vi "Set BufferLastReadsDBL.vi"(10 "BufferLastReadsDBL.lvclass":refnum<class "BufferLastReadsDBL.lvclass">, 11 "AI Current DAQmx Cont CFG in":refnum<class "AI Current DAQmx Cont CFG.lvclass">) -> (3 "AI Current DAQmx Cont CFG out":refnum<class "AI Current DAQmx Cont CFG.lvclass">)   [LabVIEW 2024, in "AI Current DAQmx Cont CFG.lvclass"]
uses:
  AI Current DAQmx Cont CFG.lvclass
  AI Current DAQmx Cont CFG.lvclass/AI Current DAQmx Cont CFG.ctl
  Buffers/BufferLastReadingsDBL/BufferLastReadsDBL.lvclass
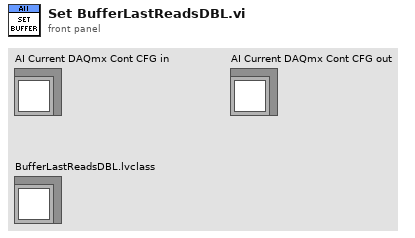
[diagram p1: front panel]
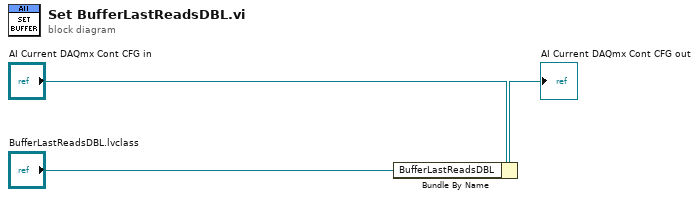
[diagram p0: block diagram]
diagram:
  n1 = Bundle By Name(cluster="AI Current DAQmx Cont CFG in", "BufferLastReadsDBL"="BufferLastReadsDBL.lvclass") -> (→"AI Current DAQmx Cont CFG out":refnum<class "AI Current DAQmx Cont CFG.lvclass">)
